vi "Update UI per Reference.vi"(8 "error in (no error)":errorcluster, 11 "Analyze Results SHG-AK in":refnum<class "Analyze Results SHG-AK.lvclass">) -> (0 "error out":errorcluster, 3 "Analyze Results SHG-AK out":refnum<class "Analyze Results SHG-AK.lvclass">)   [LabVIEW 2020, in "Analyze Results SHG-AK.lvclass"]
uses:
  Analyze Results SHG-AK.lvclass
  Analyze Results SHG-AK.lvclass/Analyze Results SHG-AK.ctl
  Results Base/Analyze Results Base.lvclass
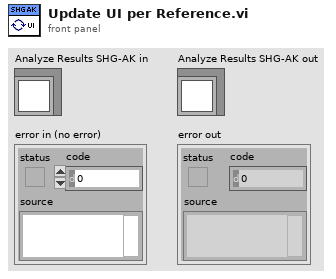
[diagram p1: front panel]
types:
  T1 = cluster{"X-Values":dbl[], "Y-ROI Averages":sgl[]}
  T2 = cluster{"X-Values":dbl[], "Gaussian Fit":dbl[]}[]
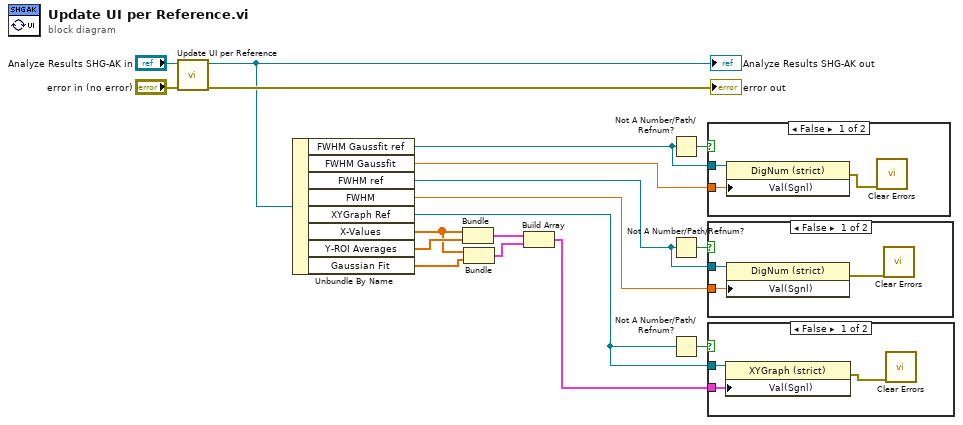
[diagram p0: block diagram]
diagram:
  n1 = call-parent "Update UI per Reference.vi"("error in (no error)"="error in (no error)", "Analyze Results Base in"="Analyze Results SHG-AK in") -> ("error out"=→"error out":errorcluster, "Analyze Results Base out"=w15:refnum<class "Analyze Results SHG-AK.lvclass">)  [unwired: 8 in]
  "Analyze Results SHG-AK out" <- w15
  n2 = Unbundle By Name(w15) -> ("FWHM Gaussfit ref"=w8:refnum<vi>, "FWHM Gaussfit"=w7:dbl[unit], "FWHM ref"=w3:refnum<vi>, "FWHM"=w1:dbl[unit], "XYGraph Ref"=w4:refnum<vi>, "X-Values"=w11:dbl[], "Y-ROI Averages"=w12:sgl[], "Gaussian Fit"=w10:dbl[])
  n3 = Bundle("X-Values"=w11, "Y-ROI Averages"=w12) -> (w13:T1)  [unwired: 1 in]
  n4 = Bundle("X-Values"=w11, "Gaussian Fit"=w10) -> (w14:cluster{"X-Values":dbl[], "Gaussian Fit":dbl[]})  [unwired: 1 in]
  n5 = Build Array(w13, w14) -> (w2:T2)
  n6 = Not A Number/Path/Refnum?(number/path/refnum=w8) -> (NaN/Path/Refnum?=w9:bool)
  n7 = Not A Number/Path/Refnum?(number/path/refnum=w3) -> (NaN/Path/Refnum?=w6:bool)
  n8 = Not A Number/Path/Refnum?(number/path/refnum=w4) -> (NaN/Path/Refnum?=w5:bool)
  n9 = case shown="False" w9 {
    tunnel: w8 -> [w21 _]
    tunnel: w7 -> [w20 _]
    frame False {
      n10 = property class="DigNum (strict)"(reference=w21, "Val(Sgnl)"=w20) -> (error out=w19:errorcluster)  [unwired: 1 in, 1 out]
      n11 = call <vilib>:"Clear Errors.vi"("error in (no error)"=w19) -> ()  [unwired: 5 in, 2 out]
    }
    frame True {
    }
  }
  n12 = case shown="False" w6 {
    tunnel: w3 -> [w24 _]
    tunnel: w1 -> [w22 _]
    frame False {
      n13 = property class="DigNum (strict)"(reference=w24, "Val(Sgnl)"=w22) -> (error out=w23:errorcluster)  [unwired: 1 in, 1 out]
      n14 = call <vilib>:"Clear Errors.vi"("error in (no error)"=w23) -> ()  [unwired: 5 in, 2 out]
    }
    frame True {
    }
  }
  n15 = case shown="False" w5 {
    tunnel: w4 -> [w27 _]
    tunnel: w2 -> [w26 _]
    frame False {
      n16 = property class="XYGraph (strict)"(reference=w27, "Val(Sgnl)"=w26) -> (error out=w25:errorcluster)  [unwired: 1 in, 1 out]
      n17 = call <vilib>:"Clear Errors.vi"("error in (no error)"=w25) -> ()  [unwired: 5 in, 2 out]
    }
    frame True {
    }
  }
